vi "Scan Module.vi"(1 "Channel":u32(ring)=1 items=["A"=1, "B"=2, "A + B"=3, "C"=4, "A + C"=5, "A + B"=6, "D"=8, "A + D"=9, "B + D"=10, "C + D"=12, "A + B + C + D"=15], 9 "Init state":T1=enum."Init(GPU FFT)", 11 "Error In":errorcluster, 12 "Start Acquire?":bool) -> (4 "Finished?":bool, 15 "Error Out":errorcluster)   [LabVIEW 2018]
uses:
  Controls/Go Scan Actions.ctl
  Controls/FGV Actions.ctl
  Controls/Queue Manager Actions.ctl
  Controls/scan status.ctl
  Hardware Mfg/Thorlabs Translation Stages/Controls/Motion Translation Module Control.ctl
  Controls/Set Get Controls.ctl
  Tile naming actions.ctl
  Hardware Mfg/AlazarTech SDK/Controls/Alazar Engine Actions.ctl
  Controls/Save Bline to Mem Control.ctl
panel:
  out "Waveform Chart":dbl(graph)
  in  "No Slice?":bool
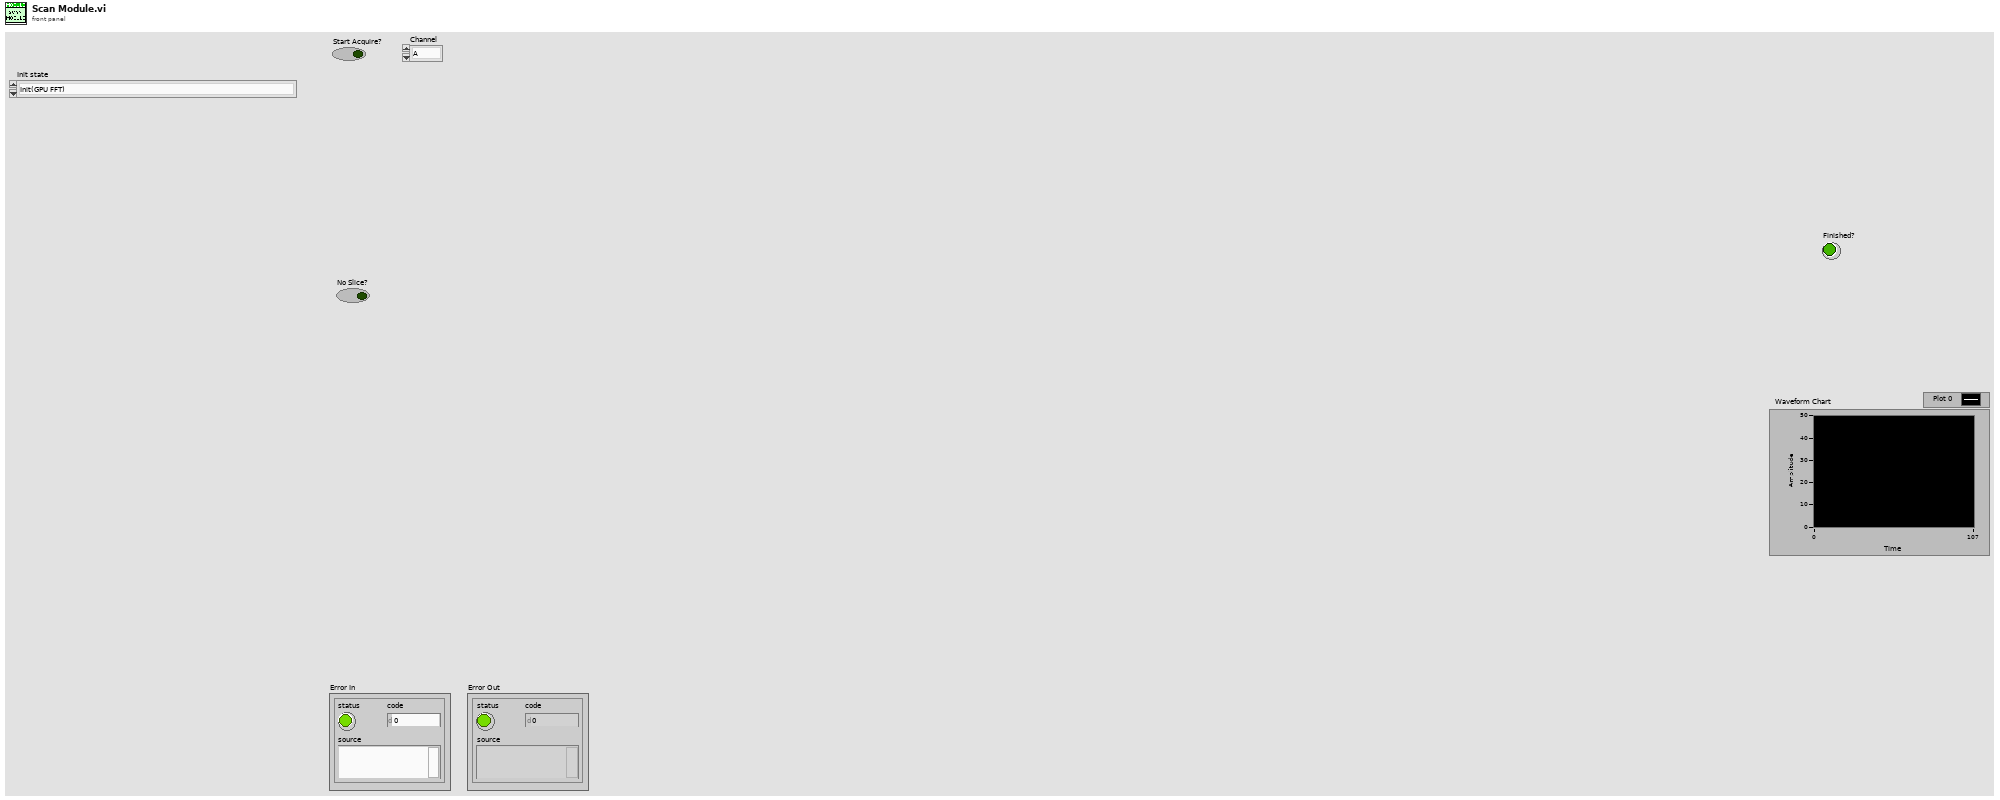
[diagram p1: front panel]
types:
  T1 = typedef "Go Scan Actions.ctl" = enum16{"Init(ThorOCT Spatial)", "Init(ThorOCT Spectral)", "Init(GPU FFT)", "Init(Alazar FFT)", "Init Scan Head(ThorOCT Spectral)", "Init Scan Head(ThorOCT Spatial)", "Init Scan Head", "Init Table Stage", "Init Vibratome", "Generate Mosaic", "Generate Z Position", "Go to Image Z", "Go Image Home", "Go Mosaic", "Acquire Image(ThorOCT Spatial)", "Acquire Image(ThorOCT Spectral)", "Acquire Image(GPU FFT)", "Acquire Image(Alazar FFT)", "Go Vibratome", "Slice", "Finished(ThorOCT)", "Finished", "Init(Alazar Spectral)"}
  T2 = typedef "FGV Actions.ctl" = enum16{"Init", "Set", "Get", "Clear"}
  T3 = typedef "System Parameters.ctl" = cluster{"Optical Parameters":T4, "Vibratome":T5, "Table Stages":T6, "Imaging Parameter":T9, "Galvo HW Parameters":cluster{"Analog Out Channel":tag, "Min Voltage":dbl, "Max Voltage":dbl, "Pixel Clock Source":tag, "Sample Rate":dbl, "Line Clock Out Ch":tag}, "Alazar parameters":T11, "Mosaic Paramter":cluster{"X Axis":cluster{"Start [mm]":dbl, "Steps [pts]":dbl, "End [mm]":dbl}, "Y Axis":cluster{"Start [mm]":dbl, "Steps [pts]":dbl, "End [mm]":dbl}, "Scan Pattern":enum16{"Uni-directional", "Bi-Directional", "Spiral Out", "Spiral In"}, "Overlap Options":cluster{"Overlap Type":enum16{"No Overlap", "X Only", "Y Only", "X and Y"}, "Percent Overlap":u8, "Justify":enum16{"Start", "Center", "End"}}}, "Manual Controls":T18, "Vibratome Axis":T21}
  T4 = typedef "Optical Parameters.ctl" = cluster{"Obj. Focal Length [mm]":dbl, "Scan Lens EFL[mm]":dbl, "Tube Lens EFL[mm]":dbl, "Galvo V Range (+/-)":dbl, "Galvo Max Half Angle [Deg]":dbl, "Max Galvo Range[%]":dbl}
  T5 = typedef "Vibratome Parameters.ctl" = cluster{"Z Bottom [mm]":dbl, "Pre Cut Dwell [s]":dbl, "Blade Frequency [RPM]":u16, "Slice Speed [mm/s]":dbl, "Post Cut Dwell [s]":dbl, "Ramp Time [s]":dbl, "Start X [mm]":dbl, "Start Y [mm]":dbl, "Slice Length [mm]":dbl, "Slice Axis":enum16{"X Axis", "Y Axis", "Z Axis"}, "Controller VISA Ref":refnum<visa-resource-name>}
  T6 = typedef "Translation Stage Parameters.ctl" = cluster{"X Stage":T7, "Y Stage":T7, "Z Stage":T7}
  T7 = typedef "Translation Stage Cluster.ctl" = cluster{"Position":dbl, "Is.Enabled?":bool, "Is.Connected?":bool, "Device SN":string, "AccelerationMaximum":dbl, "VelocityMaximum":dbl, "Acceleration":dbl, "Velocity":dbl, "waitTimeout (ms)":i32, "Model":T8, "Is.Homed?":bool}
  T8 = typedef "Translation Stage Types.ctl" = enum16{"None", "Thorlabs LTS", "Thorlabs MLJ"}
  T9 = typedef "Imaging Parameters.ctl" = cluster{"Raster Scan Direction":T10, "Pixel Dwell Time [Clock Cycles]":u16, "Flyback Time [Clock Cycles]":u16, "XY Center [um]":cluster{"X":dbl, "Y":dbl}, "Pixel Step Size [um] X":dbl, "XY Image Size":enum16{"32 x 32", "64 x 64", "128 x 128", "256 x 256", "512 x 512", "1024 x 1024", "2048 x 2048"}, "Custom":bool, "Custom Size":cluster{"X":u16, "Y":u16}, "Line Averages":u8, "Pixel Step Size [um] Y":dbl}
  T10 = typedef "Scan Direction.ctl" = enum16{"Uni Directional", "Bi Directional", "None"}
  T11 = typedef "Alazar parameters.ctl" = cluster{"Trigger Settings":cluster{"General Trigger Settings":T12, "Trigger Engine 1":T13, "Trigger Engine 2":T13}, "Device ID":T14, "Ch A Input Control":T15, "Ch B Input Control":T15, "Acq Settings":T16, "Capture Clock":T17}
  T12 = typedef "General Trigger Settings.ctl" = cluster{"Trigger Operation":u32, "Coupling ID":u32, "Range ID":u32, "Delay":u32, "Timeout Ticks":u32, "Mode":u32, "Parameter":u32}
  T13 = typedef "Trigger Engine Controls.ctl" = cluster{"Trigger Engine":u32, "Source":u32, "Slope":u32, "Level":u32}
  T14 = typedef "Alazar Device ID.ctl" = cluster{"System ID":u32, "Board ID":u32}
  T15 = typedef "Channel Input Controls.ctl" = cluster{"Channel":u8, "Coupling":u32, "Range":u32, "Impedance":u32}
  T16 = typedef "Alazar Acquisition Settings.ctl" = cluster{"Record Length":u32, "Offset":u32, "Records Per Buffer":u32, "Records Count (Records/Acq)":u32, "Window Type":u32, "Footer":u32, "Samples per record":u32, "Output Format":u32}
  T17 = typedef "Clock Controls.ctl" = cluster{"Sample Rate":u32, "Decimation":u32, "Source":u32, "Edge":u32}
  T18 = typedef "Manual Controls.ctl" = cluster{"Z0":dbl, "First image height":dbl, "Data Path":path, "Save parameters":T19, "Center Galvos":bool, "Acquisition mode":T20, "PSOCT Channel":u32, "Save":bool, "AIP rotation angle":dbl, "Scan Parameters":cluster{"# Scan":cluster{"#Ascan":i32, "#Bscan":i32}, "# Rpt":cluster{"#ARpt":i32, "#BRpt":i32}, "Aline Rate":u16, "# Extra":cluster{"# ARpt_extra":i32, "#Brtn_extra":i32}}, "ROI Parameters":cluster{"ROI (mm)":cluster{"X (mm)":dbl, "Y (mm)":dbl}, "Shift (mm)":cluster{"Xshift (mm)":sgl, "Yshift (mm)":sgl}}, "Objective":u16}
  T19 = typedef "FFT parameters.ctl" = cluster{"start pixel":i32, "#pixels to save":i32}
  T20 = typedef "FFT mode.ctl" = enum16{"ThorOCT B line", "ThorOCT Spectral", "ThorOCT FFT", "Alazar B line", "Alazar FFT", "GPU FFT", "Alazar Spectral"}
  T21 = typedef "Vibratome Param.ctl" = cluster{"Start [mm](first cut height)":dbl, "slice thickness[um]":dbl, "#slice":u16, "slice thick2[um]":dbl, "#thin slices":u16, "image thickness(um)":dbl, "#images":u16, "image depth2":dbl, "#image depth2":u16}
  T22 = typedef "Queue Manager Actions.ctl" = enum16{"Init", "Enqueue", "Enqueue All", "Preview Queue", "Dequeue", "Get Status", "Flush Queue", "Flush All Queues", "Release All Queues", "Release Queue", "Enqueue at Opposite End"}
  T23 = typedef "scan status.ctl" = enum16{"Complete Scan(ThorOCT)", "Complete Scan(PSOCT)", "Start(ThorOCT Spatial)", "Start(ThorOCT Spectral)", "Start(GPU FFT)", "Start(Alazar FFT)", "Scan(ThorOCT Spatial)", "Scan(ThorOCT Spectral)", "Scan(GPU FFT)", "Scan(Alazar FFT)", "Finish Scan(ThorOCT)", "Finish Scan(PSOCT)"}
  T24 = typedef "Set Get Controls.ctl" = enum16{"Set", "Get"}
  T25 = typedef "Motion Translation Module Control.ctl" = enum16{"Init", "Home", "Status", "Velocity/Accel", "Position", "Jog", "Stop", "Uninit", "Enable", "Disable"}
  T26 = typedef "Tile naming actions.ctl" = enum16{"Export", "Increment", "Total tile num", "Init"}
  T27 = typedef "Alazar Engine Actions.ctl" = enum16{"Init", "Config Clock", "Config Ch", "Config Trig", "Config Non-FFT Acq.", "Non-FFT Acquire", "start acquire", "Config Acq.", "Acquire", "UnInit"}
  T28 = enum16{"Configure channels", "Write Scan Pattern", "Start Galvo Task", "Is Task Done?", "Stop Galvo", "Uninit", "Init: Calc scan pattern"}
  T29 = enum16{"Init", "Configure", "Configure Data", "Generate Scan Pattern", "Start Acquire Raw", "Start Acquire Data", "Acquire RAW", "Acquire Data", "Stop Acquire", "Uninit"}
  T30 = typedef "Save Bline to Mem Control.ctl" = enum16{"Output data", "Save(ThorOCT)", "Save(PSOCT)", "FFT and Save", "Uninit", "PSOCT Spectral buffer Set", "PSOCT Spatial buffer Set", "PSOCT Spectral buffer Init", "PSOCT Spatial buffer Init", "ThorOCT Spectral buffer Init", "ThorOCT Spatial buffer Init", "ThorOCT Spectral buffer Set", "ThorOCT Spatial buffer Set", "ThorOCT Spectral Save", "Alazar Spectral Save"}
  T31 = typedef "ScanType.ctl" = enum16{"Single Frame", "Continuous Frame", "ROI Line", "Vibratome", "Mosaic", "Mosaic + Slice"}
  T32 = cluster{"X Axis":cluster{"Start [mm]":dbl, "Steps [pts]":dbl, "End [mm]":dbl}, "Y Axis":cluster{"Start [mm]":dbl, "Steps [pts]":dbl, "End [mm]":dbl}, "Scan Pattern":enum16{"Uni-directional", "Bi-Directional", "Spiral Out", "Spiral In"}, "Overlap Options":cluster{"Overlap Type":enum16{"No Overlap", "X Only", "Y Only", "X and Y"}, "Percent Overlap":u8, "Justify":enum16{"Start", "Center", "End"}}}
  T33 = cluster{"Start [mm]":dbl, "Steps [pts]":dbl, "End [mm]":dbl}
  T34 = cluster{"Overlap Type":enum16{"No Overlap", "X Only", "Y Only", "X and Y"}, "Percent Overlap":u8, "Justify":enum16{"Start", "Center", "End"}}
  T35 = enum16{"Uni-directional", "Bi-Directional", "Spiral Out", "Spiral In"}
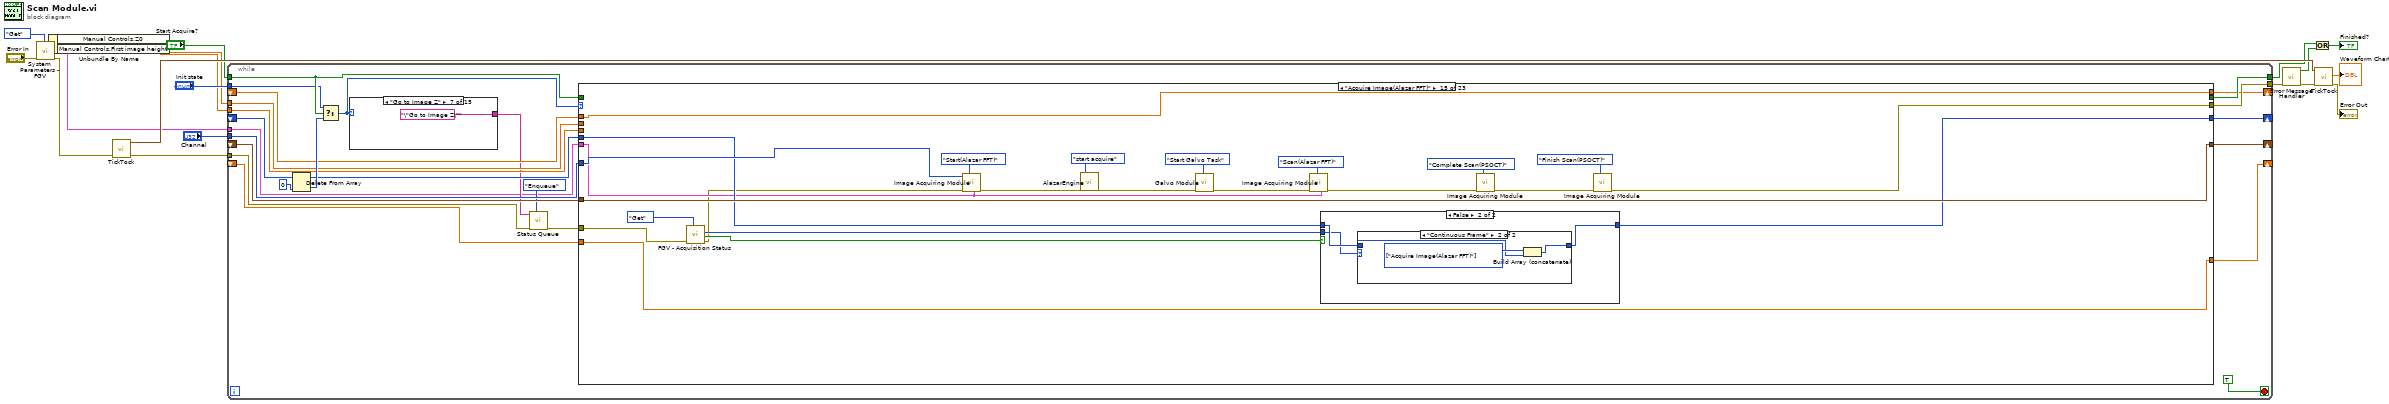
[diagram p0: block diagram]
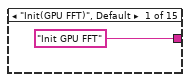
[diagram p2: hidden frame]
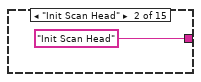
[diagram p3: hidden frame]
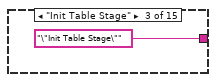
[diagram p4: hidden frame]
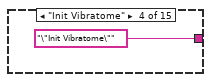
[diagram p5: hidden frame]
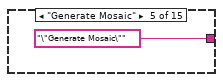
[diagram p6: hidden frame]
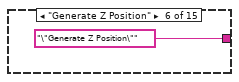
[diagram p7: hidden frame]
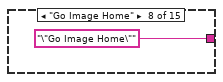
[diagram p8: hidden frame]
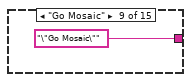
[diagram p9: hidden frame]
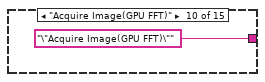
[diagram p10: hidden frame]
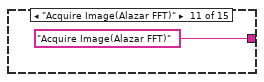
[diagram p11: hidden frame]
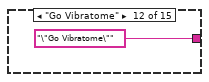
[diagram p12: hidden frame]
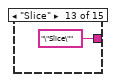
[diagram p13: hidden frame]
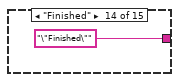
[diagram p14: hidden frame]
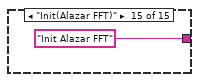
[diagram p15: hidden frame]
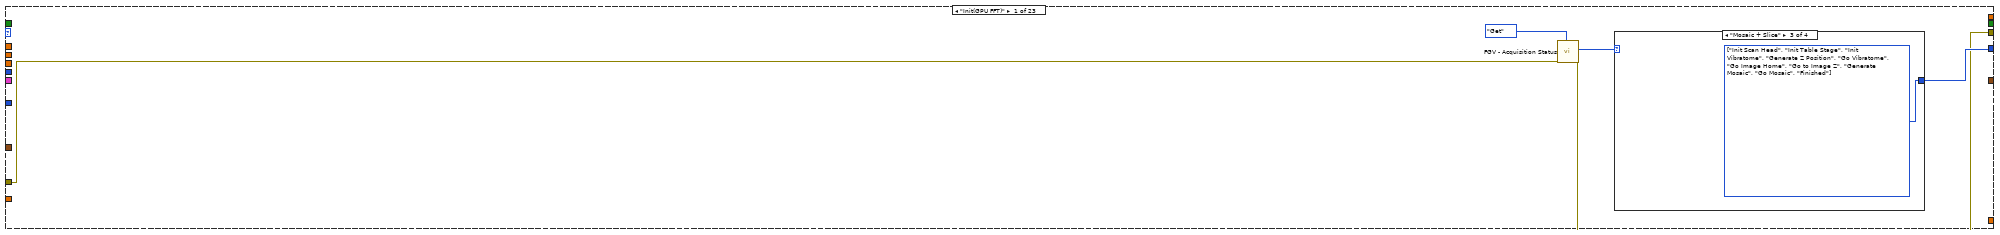
[diagram p16: hidden frame]
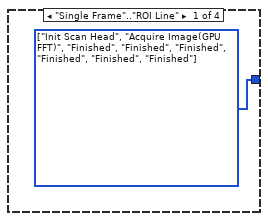
[diagram p17: hidden frame]
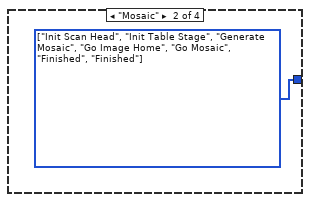
[diagram p18: hidden frame]
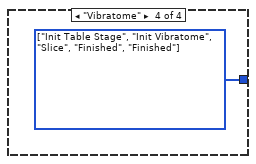
[diagram p19: hidden frame]
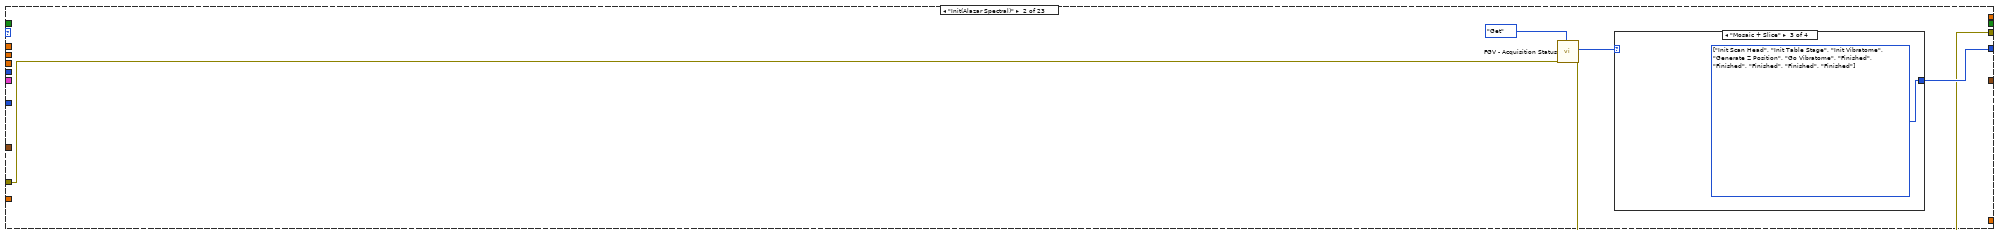
[diagram p20: hidden frame]
diagram:
  n1 = call "System Parameters - FGV.vi"("Actions"=FGV_Actions."Get", "Error In"="Error In") -> ("Error Out"=w4:errorcluster, "System Parameters [Out]"=w3:T3)  [unwired: 8 in]
  n2 = Unbundle By Name(w3) -> ("Manual Controls.Z0"=w2:dbl, "Manual Controls.First image height"=w1:dbl)
  n3 = call "TickTock.vi"("Error In"=w4) -> ("Error Out"=w16:errorcluster, "Current Time (Out)"=w14:timestamp)  [unwired: 8 in, 1 out]
  n4 = while {
    shift-right: [w37] -> _
    shift-left: _ -> [w42]
    tunnel: "Start Acquire?" -> [w38]
    shift-right: [w36] -> _
    shift-left: _ -> [w34]
    tunnel: w16 -> [w24]
    tunnel: [w35] -> w18
    tunnel: [w33] -> w10
    tunnel: w1 -> [w32]
    shift-right: [w30] -> _
    shift-left: _ -> [w28]
    shift-right: [w31] -> _
    shift-left: _ -> [w29]
    tunnel: "Init state" -> [w27]
    tunnel: w2 -> [w26]
    tunnel: "Channel" -> [w25]
    tunnel: w3 -> [w19]
    stop <- TRUE stop-if-true
    n5 = Delete From Array(array=w42, index=0) -> (deleted portion=w41:T1, array with subset deleted=w40:T1[])  [unwired: 1 in]
    n6 = Select(t=w27, s=w38, f=w41) -> (s? t:f=w22:T1)
    n7 = case shown="\"Go to Image Z\"" w22 {
      tunnel: ["Init GPU FFT" "Init Scan Head" "\"Init Table Stage\"" "\"Init Vibratome\"" "\"Generate Mosaic\"" "\"Generate Z Position\"" "\"Go to Image Z\"" "\"Go Image Home\"" "\"Go Mosaic\"" "\"Acquire Image(GPU FFT)\"" "Acquire Image(Alazar FFT)" "\"Go Vibratome\"" "\"Slice\"" "\"Finished\"" "Init Alazar FFT"] -> w21
      frame "Init(GPU FFT)", Default {
      }
      frame "Init Scan Head" {
      }
      frame "Init Table Stage" {
      }
      frame "Init Vibratome" {
      }
      frame "Generate Mosaic" {
      }
      frame "Generate Z Position" {
      }
      frame "Go to Image Z" {
      }
      frame "Go Image Home" {
      }
      frame "Go Mosaic" {
      }
      frame "Acquire Image(GPU FFT)" {
      }
      frame "Acquire Image(Alazar FFT)" {
      }
      frame "Go Vibratome" {
      }
      frame "Slice" {
      }
      frame "Finished" {
      }
      frame "Init(Alazar FFT)" {
      }
    }
    n8 = call "Status Queue.vi"("Action"=Queue_Manager_Actions."Enqueue", "Error In"=w24, "Status Message [In]"=w21) -> ("Error Out"=w23:errorcluster)  [unwired: 7 in, 1 out]
    n9 = case shown="\"Acquire Image(Alazar FFT)\"" w22 {
      selector: w22 -> [_ _ _ _ _ _ _ _ _ _ _ _ _ _ _ _ _ _ w397 _ _ _ _]
      tunnel: [w62 w71 w80 w89 w97 w118 w125 w133 w141 w172 w182 w198 w220 w232 w279 w311 w336 w364 w403 w465 w530 _ _] -> w37
      tunnel: w40 -> [_ _ _ _ _ w118 w125 w133 w141 w172 w182 w198 w220 w233 w282 w314 w339 w365 w405 w467 w532 _ _]
      tunnel: [_ _ _ _ _ w121 w126 w134 w142 w173 w183 w185 w231 w241 w295 w320 w345 w370 w406 w468 w533 _ _] -> w36
      tunnel: w34 -> [_ _ _ _ _ w121 w126 w134 w142 w173 w183 _ w231 w241 w295 w320 w345 w370 w402 w468 w533 _ _]
      tunnel: [w59 w68 w77 w86 w95 w119 w122 w129 w137 w171 w177 w186 w214 w240 w277 w305 w330 w358 w404 w466 w531 w550 w594] -> w35
      tunnel: w38 -> [_ _ _ _ _ _ _ _ _ _ _ _ _ _ _ _ _ _ _ _ _ _ _]
      tunnel: [_ _ _ _ _ _ _ _ _ _ _ _ _ _ _ _ _ _ _ _ w524 TRUE TRUE] -> w33
      tunnel: w32 -> [_ _ _ _ _ w111 _ _ _ _ _ _ _ _ _ _ _ _ _ _ _ _ _]
      tunnel: [_ _ _ _ _ w116 w123 w131 w139 w169 w181 w192 w216 w238 w286 w317 w342 w368 w395 w459 w523 _ _] -> w31
      tunnel: [_ _ _ _ _ w110 w124 w132 w140 w170 w180 w191 w215 w236 w285 w316 w341 w367 w393 w458 w527 _ _] -> w30
      tunnel: w29 -> [_ _ _ _ _ _ w123 w131 w139 w169 w181 w192 w216 w238 w286 w317 w342 w368 w395 w456 w523 _ _]
      tunnel: w28 -> [_ _ _ _ _ _ w124 w132 w140 w170 w180 w191 w215 w234 w285 w316 w341 w367 w393 w458 w527 _ _]
      tunnel: w23 -> [w60 w69 w78 w87 w96 w119 w122 w130 w138 w144 w178 w190 w200 w237 w275 w308 w333 w362 w394 w464 w529 w551 w595]
      tunnel: w26 -> [_ _ _ _ _ _ _ _ _ _ _ _ _ _ _ _ _ _ _ w463 w528 _ _]
      tunnel: w25 -> [_ _ _ _ _ _ _ _ _ _ _ _ _ _ w283 _ _ w366 _ _ _ _ _]
      tunnel: w19 -> [_ _ _ _ _ w120 _ w128 w136 w143 w176 w189 w199 w239 w273 w309 w334 w359 w396 w457 w526 w563 w607]
      frame "Init(GPU FFT)" {
        n10 = call "FGV - Acquisition Status.vi"("Actions"=FGV_Actions."Get", "Error In"=w60) -> ("Error Out"=w59:errorcluster, "Scan Type [Out]"=w61:T31)  [unwired: 5 in, 3 out]
        n11 = case shown="\"Mosaic + Slice\"" w61 {
          tunnel: [w64 w65 w66 w67] -> w62
          frame "Single Frame".."ROI Line" {
            w64 = T1[] [enum."Init Scan Head", enum."Acquire Image(GPU FFT)", enum."Finished", enum."Finished", enum."Finished", enum."Finished", enum."Finished", enum."Finished"] items=["Init(ThorOCT Spatial)", "Init(ThorOCT Spectral)", "Init(GPU FFT)", "Init(Alazar FFT)", "Init Scan Head(ThorOCT Spectral)", "Init Scan Head(ThorOCT Spatial)", "Init Scan Head", "Init Table Stage", "Init Vibratome", "Generate Mosaic", "Generate Z Position", "Go to Image Z", "Go Image Home", "Go Mosaic", "Acquire Image(ThorOCT Spatial)", "Acquire Image(ThorOCT Spectral)", "Acquire Image(GPU FFT)", "Acquire Image(Alazar FFT)", "Go Vibratome", "Slice", "Finished(ThorOCT)", "Finished", "Init(Alazar Spectral)"]
          }
          frame "Mosaic" {
            w65 = T1[] [enum."Init Scan Head", enum."Init Table Stage", enum."Generate Mosaic", enum."Go Image Home", enum."Go Mosaic", enum."Finished", enum."Finished"] items=["Init(ThorOCT Spatial)", "Init(ThorOCT Spectral)", "Init(GPU FFT)", "Init(Alazar FFT)", "Init Scan Head(ThorOCT Spectral)", "Init Scan Head(ThorOCT Spatial)", "Init Scan Head", "Init Table Stage", "Init Vibratome", "Generate Mosaic", "Generate Z Position", "Go to Image Z", "Go Image Home", "Go Mosaic", "Acquire Image(ThorOCT Spatial)", "Acquire Image(ThorOCT Spectral)", "Acquire Image(GPU FFT)", "Acquire Image(Alazar FFT)", "Go Vibratome", "Slice", "Finished(ThorOCT)", "Finished", "Init(Alazar Spectral)"]
          }
          frame "Mosaic + Slice" {
            w66 = T1[] [enum."Init Scan Head", enum."Init Table Stage", enum."Init Vibratome", enum."Generate Z Position", enum."Go Vibratome", enum."Go Image Home", enum."Go to Image Z", enum."Generate Mosaic", enum."Go Mosaic", enum."Finished"] items=["Init(ThorOCT Spatial)", "Init(ThorOCT Spectral)", "Init(GPU FFT)", "Init(Alazar FFT)", "Init Scan Head(ThorOCT Spectral)", "Init Scan Head(ThorOCT Spatial)", "Init Scan Head", "Init Table Stage", "Init Vibratome", "Generate Mosaic", "Generate Z Position", "Go to Image Z", "Go Image Home", "Go Mosaic", "Acquire Image(ThorOCT Spatial)", "Acquire Image(ThorOCT Spectral)", "Acquire Image(GPU FFT)", "Acquire Image(Alazar FFT)", "Go Vibratome", "Slice", "Finished(ThorOCT)", "Finished", "Init(Alazar Spectral)"]
          }
          frame "Vibratome" {
            w67 = T1[] [enum."Init Table Stage", enum."Init Vibratome", enum."Slice", enum."Finished", enum."Finished"] items=["Init(ThorOCT Spatial)", "Init(ThorOCT Spectral)", "Init(GPU FFT)", "Init(Alazar FFT)", "Init Scan Head(ThorOCT Spectral)", "Init Scan Head(ThorOCT Spatial)", "Init Scan Head", "Init Table Stage", "Init Vibratome", "Generate Mosaic", "Generate Z Position", "Go to Image Z", "Go Image Home", "Go Mosaic", "Acquire Image(ThorOCT Spatial)", "Acquire Image(ThorOCT Spectral)", "Acquire Image(GPU FFT)", "Acquire Image(Alazar FFT)", "Go Vibratome", "Slice", "Finished(ThorOCT)", "Finished", "Init(Alazar Spectral)"]
          }
        }
      }
      frame "Init(Alazar Spectral)" {
        n12 = call "FGV - Acquisition Status.vi"("Actions"=FGV_Actions."Get", "Error In"=w69) -> ("Error Out"=w68:errorcluster, "Scan Type [Out]"=w70:T31)  [unwired: 5 in, 3 out]
        n13 = case shown="\"Mosaic + Slice\"" w70 {
          tunnel: [w73 w74 w75 w76] -> w71
          frame "Single Frame".."ROI Line" {
            w73 = T1[] [enum."Init Scan Head", enum."Init Scan Head", enum."Acquire Image(GPU FFT)", enum."Finished", enum."Acquire Image(GPU FFT)", enum."Finished", enum."Acquire Image(GPU FFT)", enum."Finished"] items=["Init(ThorOCT Spatial)", "Init(ThorOCT Spectral)", "Init(GPU FFT)", "Init(Alazar FFT)", "Init Scan Head(ThorOCT Spectral)", "Init Scan Head(ThorOCT Spatial)", "Init Scan Head", "Init Table Stage", "Init Vibratome", "Generate Mosaic", "Generate Z Position", "Go to Image Z", "Go Image Home", "Go Mosaic", "Acquire Image(ThorOCT Spatial)", "Acquire Image(ThorOCT Spectral)", "Acquire Image(GPU FFT)", "Acquire Image(Alazar FFT)", "Go Vibratome", "Slice", "Finished(ThorOCT)", "Finished", "Init(Alazar Spectral)"]
          }
          frame "Mosaic" {
            w74 = T1[] [enum."Init Scan Head", enum."Init Table Stage", enum."Generate Mosaic", enum."Go Image Home", enum."Go Mosaic", enum."Finished", enum."Finished"] items=["Init(ThorOCT Spatial)", "Init(ThorOCT Spectral)", "Init(GPU FFT)", "Init(Alazar FFT)", "Init Scan Head(ThorOCT Spectral)", "Init Scan Head(ThorOCT Spatial)", "Init Scan Head", "Init Table Stage", "Init Vibratome", "Generate Mosaic", "Generate Z Position", "Go to Image Z", "Go Image Home", "Go Mosaic", "Acquire Image(ThorOCT Spatial)", "Acquire Image(ThorOCT Spectral)", "Acquire Image(GPU FFT)", "Acquire Image(Alazar FFT)", "Go Vibratome", "Slice", "Finished(ThorOCT)", "Finished", "Init(Alazar Spectral)"]
          }
          frame "Mosaic + Slice" {
            w75 = T1[] [enum."Init Scan Head", enum."Init Table Stage", enum."Init Vibratome", enum."Generate Z Position", enum."Go Vibratome", enum."Finished", enum."Finished", enum."Finished", enum."Finished", enum."Finished"] items=["Init(ThorOCT Spatial)", "Init(ThorOCT Spectral)", "Init(GPU FFT)", "Init(Alazar FFT)", "Init Scan Head(ThorOCT Spectral)", "Init Scan Head(ThorOCT Spatial)", "Init Scan Head", "Init Table Stage", "Init Vibratome", "Generate Mosaic", "Generate Z Position", "Go to Image Z", "Go Image Home", "Go Mosaic", "Acquire Image(ThorOCT Spatial)", "Acquire Image(ThorOCT Spectral)", "Acquire Image(GPU FFT)", "Acquire Image(Alazar FFT)", "Go Vibratome", "Slice", "Finished(ThorOCT)", "Finished", "Init(Alazar Spectral)"]
          }
          frame "Vibratome" {
            w76 = T1[] [enum."Init Table Stage", enum."Init Vibratome", enum."Slice", enum."Finished", enum."Finished"] items=["Init(ThorOCT Spatial)", "Init(ThorOCT Spectral)", "Init(GPU FFT)", "Init(Alazar FFT)", "Init Scan Head(ThorOCT Spectral)", "Init Scan Head(ThorOCT Spatial)", "Init Scan Head", "Init Table Stage", "Init Vibratome", "Generate Mosaic", "Generate Z Position", "Go to Image Z", "Go Image Home", "Go Mosaic", "Acquire Image(ThorOCT Spatial)", "Acquire Image(ThorOCT Spectral)", "Acquire Image(GPU FFT)", "Acquire Image(Alazar FFT)", "Go Vibratome", "Slice", "Finished(ThorOCT)", "Finished", "Init(Alazar Spectral)"]
          }
        }
      }
      frame "Init(ThorOCT Spatial)" {
        n14 = call "FGV - Acquisition Status.vi"("Actions"=FGV_Actions."Get", "Error In"=w78) -> ("Error Out"=w77:errorcluster, "Scan Type [Out]"=w79:T31)  [unwired: 5 in, 3 out]
        n15 = case shown="\"Single Frame\"..\"ROI Line\"" w79 {
          tunnel: [w82 w83 w84 w85] -> w80
          frame "Single Frame".."ROI Line" {
            w82 = T1[] [enum."Init Scan Head(ThorOCT Spatial)", enum."Acquire Image(ThorOCT Spatial)", enum."Finished(ThorOCT)", enum."Finished", enum."Acquire Image(GPU FFT)", enum."Finished", enum."Acquire Image(GPU FFT)", enum."Finished"] items=["Init(ThorOCT Spatial)", "Init(ThorOCT Spectral)", "Init(GPU FFT)", "Init(Alazar FFT)", "Init Scan Head(ThorOCT Spectral)", "Init Scan Head(ThorOCT Spatial)", "Init Scan Head", "Init Table Stage", "Init Vibratome", "Generate Mosaic", "Generate Z Position", "Go to Image Z", "Go Image Home", "Go Mosaic", "Acquire Image(ThorOCT Spatial)", "Acquire Image(ThorOCT Spectral)", "Acquire Image(GPU FFT)", "Acquire Image(Alazar FFT)", "Go Vibratome", "Slice", "Finished(ThorOCT)", "Finished", "Init(Alazar Spectral)"]
          }
          frame "Mosaic" {
            w83 = T1[] [enum."Init Scan Head(ThorOCT Spatial)", enum."Init Table Stage", enum."Generate Mosaic", enum."Go Image Home", enum."Go Mosaic", enum."Finished(ThorOCT)", enum."Finished"] items=["Init(ThorOCT Spatial)", "Init(ThorOCT Spectral)", "Init(GPU FFT)", "Init(Alazar FFT)", "Init Scan Head(ThorOCT Spectral)", "Init Scan Head(ThorOCT Spatial)", "Init Scan Head", "Init Table Stage", "Init Vibratome", "Generate Mosaic", "Generate Z Position", "Go to Image Z", "Go Image Home", "Go Mosaic", "Acquire Image(ThorOCT Spatial)", "Acquire Image(ThorOCT Spectral)", "Acquire Image(GPU FFT)", "Acquire Image(Alazar FFT)", "Go Vibratome", "Slice", "Finished(ThorOCT)", "Finished", "Init(Alazar Spectral)"]
          }
          frame "Mosaic + Slice" {
            w84 = T1[] [enum."Init Scan Head(ThorOCT Spatial)", enum."Init Table Stage", enum."Init Vibratome", enum."Generate Z Position", enum."Generate Mosaic", enum."Go Image Home", enum."Go Mosaic", enum."Go Vibratome", enum."Finished(ThorOCT)", enum."Finished"] items=["Init(ThorOCT Spatial)", "Init(ThorOCT Spectral)", "Init(GPU FFT)", "Init(Alazar FFT)", "Init Scan Head(ThorOCT Spectral)", "Init Scan Head(ThorOCT Spatial)", "Init Scan Head", "Init Table Stage", "Init Vibratome", "Generate Mosaic", "Generate Z Position", "Go to Image Z", "Go Image Home", "Go Mosaic", "Acquire Image(ThorOCT Spatial)", "Acquire Image(ThorOCT Spectral)", "Acquire Image(GPU FFT)", "Acquire Image(Alazar FFT)", "Go Vibratome", "Slice", "Finished(ThorOCT)", "Finished", "Init(Alazar Spectral)"]
          }
          frame "Vibratome" {
            w85 = T1[] [enum."Init Table Stage", enum."Init Vibratome", enum."Slice", enum."Finished(ThorOCT)", enum."Finished(ThorOCT)"] items=["Init(ThorOCT Spatial)", "Init(ThorOCT Spectral)", "Init(GPU FFT)", "Init(Alazar FFT)", "Init Scan Head(ThorOCT Spectral)", "Init Scan Head(ThorOCT Spatial)", "Init Scan Head", "Init Table Stage", "Init Vibratome", "Generate Mosaic", "Generate Z Position", "Go to Image Z", "Go Image Home", "Go Mosaic", "Acquire Image(ThorOCT Spatial)", "Acquire Image(ThorOCT Spectral)", "Acquire Image(GPU FFT)", "Acquire Image(Alazar FFT)", "Go Vibratome", "Slice", "Finished(ThorOCT)", "Finished", "Init(Alazar Spectral)"]
          }
        }
      }
      frame "Init(ThorOCT Spectral)" {
        n16 = call "FGV - Acquisition Status.vi"("Actions"=FGV_Actions."Get", "Error In"=w87) -> ("Error Out"=w86:errorcluster, "Scan Type [Out]"=w88:T31)  [unwired: 5 in, 3 out]
        n17 = case shown="\"Vibratome\"" w88 {
          tunnel: [w91 w92 w93 w94] -> w89
          frame "Single Frame".."ROI Line" {
            w91 = T1[] [enum."Init Scan Head(ThorOCT Spectral)", enum."Acquire Image(ThorOCT Spectral)", enum."Finished(ThorOCT)", enum."Finished", enum."Acquire Image(GPU FFT)", enum."Finished", enum."Acquire Image(GPU FFT)", enum."Finished"] items=["Init(ThorOCT Spatial)", "Init(ThorOCT Spectral)", "Init(GPU FFT)", "Init(Alazar FFT)", "Init Scan Head(ThorOCT Spectral)", "Init Scan Head(ThorOCT Spatial)", "Init Scan Head", "Init Table Stage", "Init Vibratome", "Generate Mosaic", "Generate Z Position", "Go to Image Z", "Go Image Home", "Go Mosaic", "Acquire Image(ThorOCT Spatial)", "Acquire Image(ThorOCT Spectral)", "Acquire Image(GPU FFT)", "Acquire Image(Alazar FFT)", "Go Vibratome", "Slice", "Finished(ThorOCT)", "Finished", "Init(Alazar Spectral)"]
          }
          frame "Mosaic" {
            w92 = T1[] [enum."Init Scan Head(ThorOCT Spectral)", enum."Init Table Stage", enum."Generate Mosaic", enum."Go Image Home", enum."Go Mosaic", enum."Finished(ThorOCT)", enum."Finished"] items=["Init(ThorOCT Spatial)", "Init(ThorOCT Spectral)", "Init(GPU FFT)", "Init(Alazar FFT)", "Init Scan Head(ThorOCT Spectral)", "Init Scan Head(ThorOCT Spatial)", "Init Scan Head", "Init Table Stage", "Init Vibratome", "Generate Mosaic", "Generate Z Position", "Go to Image Z", "Go Image Home", "Go Mosaic", "Acquire Image(ThorOCT Spatial)", "Acquire Image(ThorOCT Spectral)", "Acquire Image(GPU FFT)", "Acquire Image(Alazar FFT)", "Go Vibratome", "Slice", "Finished(ThorOCT)", "Finished", "Init(Alazar Spectral)"]
          }
          frame "Mosaic + Slice" {
            w93 = T1[] [enum."Init Scan Head(ThorOCT Spectral)", enum."Init Table Stage", enum."Init Vibratome", enum."Generate Z Position", enum."Generate Mosaic", enum."Go Image Home", enum."Go Mosaic", enum."Go Vibratome", enum."Finished(ThorOCT)", enum."Finished"] items=["Init(ThorOCT Spatial)", "Init(ThorOCT Spectral)", "Init(GPU FFT)", "Init(Alazar FFT)", "Init Scan Head(ThorOCT Spectral)", "Init Scan Head(ThorOCT Spatial)", "Init Scan Head", "Init Table Stage", "Init Vibratome", "Generate Mosaic", "Generate Z Position", "Go to Image Z", "Go Image Home", "Go Mosaic", "Acquire Image(ThorOCT Spatial)", "Acquire Image(ThorOCT Spectral)", "Acquire Image(GPU FFT)", "Acquire Image(Alazar FFT)", "Go Vibratome", "Slice", "Finished(ThorOCT)", "Finished", "Init(Alazar Spectral)"]
          }
          frame "Vibratome" {
            w94 = T1[] [enum."Init Table Stage", enum."Init Vibratome", enum."Slice", enum."Finished(ThorOCT)", enum."Finished(ThorOCT)"] items=["Init(ThorOCT Spatial)", "Init(ThorOCT Spectral)", "Init(GPU FFT)", "Init(Alazar FFT)", "Init Scan Head(ThorOCT Spectral)", "Init Scan Head(ThorOCT Spatial)", "Init Scan Head", "Init Table Stage", "Init Vibratome", "Generate Mosaic", "Generate Z Position", "Go to Image Z", "Go Image Home", "Go Mosaic", "Acquire Image(ThorOCT Spatial)", "Acquire Image(ThorOCT Spectral)", "Acquire Image(GPU FFT)", "Acquire Image(Alazar FFT)", "Go Vibratome", "Slice", "Finished(ThorOCT)", "Finished", "Init(Alazar Spectral)"]
          }
        }
      }
      frame "Init(Alazar FFT)" {
        n18 = call "FGV - Acquisition Status.vi"("Actions"=FGV_Actions."Get", "Error In"=w96) -> ("Error Out"=w95:errorcluster, "Scan Type [Out]"=w98:T31)  [unwired: 5 in, 3 out]
        n19 = case shown="\"Mosaic + Slice\"" w98 {
          tunnel: [w100 w101 w102 w103 w104] -> w97
          frame "Single Frame", Default {
            w100 = T1[] [enum."Init Scan Head", enum."Acquire Image(Alazar FFT)", enum."Finished", enum."Finished", enum."Acquire Image(Alazar FFT)", enum."Finished", enum."Acquire Image(Alazar FFT)", enum."Finished"] items=["Init(ThorOCT Spatial)", "Init(ThorOCT Spectral)", "Init(GPU FFT)", "Init(Alazar FFT)", "Init Scan Head(ThorOCT Spectral)", "Init Scan Head(ThorOCT Spatial)", "Init Scan Head", "Init Table Stage", "Init Vibratome", "Generate Mosaic", "Generate Z Position", "Go to Image Z", "Go Image Home", "Go Mosaic", "Acquire Image(ThorOCT Spatial)", "Acquire Image(ThorOCT Spectral)", "Acquire Image(GPU FFT)", "Acquire Image(Alazar FFT)", "Go Vibratome", "Slice", "Finished(ThorOCT)", "Finished", "Init(Alazar Spectral)"]
          }
          frame "Continuous Frame" {
            w101 = T1[] [enum."Init Scan Head", enum."Acquire Image(Alazar FFT)", enum."Finished", enum."Finished", enum."Acquire Image(Alazar FFT)", enum."Finished", enum."Acquire Image(Alazar FFT)", enum."Finished"] items=["Init(ThorOCT Spatial)", "Init(ThorOCT Spectral)", "Init(GPU FFT)", "Init(Alazar FFT)", "Init Scan Head(ThorOCT Spectral)", "Init Scan Head(ThorOCT Spatial)", "Init Scan Head", "Init Table Stage", "Init Vibratome", "Generate Mosaic", "Generate Z Position", "Go to Image Z", "Go Image Home", "Go Mosaic", "Acquire Image(ThorOCT Spatial)", "Acquire Image(ThorOCT Spectral)", "Acquire Image(GPU FFT)", "Acquire Image(Alazar FFT)", "Go Vibratome", "Slice", "Finished(ThorOCT)", "Finished", "Init(Alazar Spectral)"]
          }
          frame "Mosaic" {
            w102 = T1[] [enum."Init Scan Head", enum."Init Table Stage", enum."Generate Mosaic", enum."Go Image Home", enum."Go Mosaic", enum."Finished", enum."Finished"] items=["Init(ThorOCT Spatial)", "Init(ThorOCT Spectral)", "Init(GPU FFT)", "Init(Alazar FFT)", "Init Scan Head(ThorOCT Spectral)", "Init Scan Head(ThorOCT Spatial)", "Init Scan Head", "Init Table Stage", "Init Vibratome", "Generate Mosaic", "Generate Z Position", "Go to Image Z", "Go Image Home", "Go Mosaic", "Acquire Image(ThorOCT Spatial)", "Acquire Image(ThorOCT Spectral)", "Acquire Image(GPU FFT)", "Acquire Image(Alazar FFT)", "Go Vibratome", "Slice", "Finished(ThorOCT)", "Finished", "Init(Alazar Spectral)"]
          }
          frame "Mosaic + Slice" {
            w103 = T1[] [enum."Init Scan Head", enum."Init Table Stage", enum."Init Vibratome", enum."Generate Z Position", enum."Go Vibratome", enum."Finished"] items=["Init(ThorOCT Spatial)", "Init(ThorOCT Spectral)", "Init(GPU FFT)", "Init(Alazar FFT)", "Init Scan Head(ThorOCT Spectral)", "Init Scan Head(ThorOCT Spatial)", "Init Scan Head", "Init Table Stage", "Init Vibratome", "Generate Mosaic", "Generate Z Position", "Go to Image Z", "Go Image Home", "Go Mosaic", "Acquire Image(ThorOCT Spatial)", "Acquire Image(ThorOCT Spectral)", "Acquire Image(GPU FFT)", "Acquire Image(Alazar FFT)", "Go Vibratome", "Slice", "Finished(ThorOCT)", "Finished", "Init(Alazar Spectral)"]
          }
          frame "Vibratome" {
            w104 = T1[] [enum."Init Table Stage", enum."Init Vibratome", enum."Slice", enum."Finished", enum."Finished"] items=["Init(ThorOCT Spatial)", "Init(ThorOCT Spectral)", "Init(GPU FFT)", "Init(Alazar FFT)", "Init Scan Head(ThorOCT Spectral)", "Init Scan Head(ThorOCT Spatial)", "Init Scan Head", "Init Table Stage", "Init Vibratome", "Generate Mosaic", "Generate Z Position", "Go to Image Z", "Go Image Home", "Go Mosaic", "Acquire Image(ThorOCT Spatial)", "Acquire Image(ThorOCT Spectral)", "Acquire Image(GPU FFT)", "Acquire Image(Alazar FFT)", "Go Vibratome", "Slice", "Finished(ThorOCT)", "Finished", "Init(Alazar Spectral)"]
          }
        }
      }
      frame "Generate Z Position" {
        w109 = 0.0
        w113 = 0.0 ("y")
        n20 = Unbundle By Name(w120) -> ("Vibratome Axis"=w117:T21)
        n21 = Unbundle By Name(w117) -> ("image thickness(um)"=w107:dbl, "#images"=w105:u16)
        n22 = Unbundle By Name(w117) -> ("Start [mm](first cut height)"=w115:dbl, "slice thickness[um]"=w114:dbl, "#slice"=w112:u16)
        n23 = Multiply(x=w112, y=w105) -> (x*y=w106:u16)
        n24 = call "Generate Z stage Position Aarray.vi"("#rep1"=w106, "#rep2"=w113, "thickness2"=w113, "Start Z"=w115, "thickness1"=w114) -> ("Array"=w116:dbl[])  [unwired: 6 in]
        n25 = Decrement(x=w105) -> (x-1=w108:u16)
        n26 = call "Generate Z stage Position Aarray.vi"("#rep1"=w108, "#rep2"=w109, "thickness2"=w109, "Start Z"=w111, "thickness1"=w107) -> ("Array"=w110:dbl[])  [unwired: 6 in]
      }
      frame "Init Scan Head" {
      }
      frame "Init Scan Head(ThorOCT Spatial)" {
        n27 = call "Image Acquiring Module.vi"("System Parameters"=w128, "Scan Status in"=scan_status."Start(ThorOCT Spatial)" ("Scan Status in 2"), "Error in"=w130) -> ("Error Out"=w129:errorcluster)  [unwired: 8 in]
      }
      frame "Init Scan Head(ThorOCT Spectral)" {
        n28 = call "Image Acquiring Module.vi"("System Parameters"=w136, "Scan Status in"=scan_status."Start(ThorOCT Spectral)" ("Scan Status in 2"), "Error in"=w138) -> ("Error Out"=w137:errorcluster)  [unwired: 8 in]
      }
      frame "Init Table Stage" {
        n29 = Unbundle By Name(w143) -> ("Table Stages"=w145:T6)
        n30 = call "XYZ Table Stage Module.vi"("Set/Get"=Set_Get_Controls."Set", "Action"=Motion_Translation_Module_Control."Init", "Error In"=w144, "Axis"=enum16{"X Axis", "Y Axis", "Z Axis"}."X Axis", "Table Stages"=w145) -> ("Error Out"=w167:errorcluster)  [unwired: 5 in, 1 out]
        n31 = call "XYZ Table Stage Module.vi"("Set/Get"=Set_Get_Controls."Set", "Action"=Motion_Translation_Module_Control."Init", "Error In"=w167, "Axis"=enum16{"X Axis", "Y Axis", "Z Axis"}."Y Axis", "Table Stages"=w145) -> ("Error Out"=w160:errorcluster)  [unwired: 5 in, 1 out]
        n32 = call "XYZ Table Stage Module.vi"("Set/Get"=Set_Get_Controls."Set", "Action"=Motion_Translation_Module_Control."Init", "Error In"=w160, "Axis"=enum16{"X Axis", "Y Axis", "Z Axis"}."Z Axis", "Table Stages"=w145) -> ("Error Out"=w146:errorcluster)  [unwired: 5 in, 1 out]
        n33 = call "XYZ Table Stage Module.vi"("Set/Get"=Set_Get_Controls."Set", "Action"=Motion_Translation_Module_Control."Velocity/Accel", "Error In"=w146, "Axis"=enum16{"X Axis", "Y Axis", "Z Axis"}."X Axis", "Table Stages"=w145) -> ("Error Out"=w156:errorcluster)  [unwired: 5 in, 1 out]
        n34 = call "XYZ Table Stage Module.vi"("Set/Get"=Set_Get_Controls."Set", "Action"=Motion_Translation_Module_Control."Velocity/Accel", "Error In"=w156, "Axis"=enum16{"X Axis", "Y Axis", "Z Axis"}."Y Axis", "Table Stages"=w145) -> ("Error Out"=w149:errorcluster)  [unwired: 5 in, 1 out]
        n35 = call "XYZ Table Stage Module.vi"("Set/Get"=Set_Get_Controls."Set", "Action"=Motion_Translation_Module_Control."Velocity/Accel", "Error In"=w149, "Axis"=enum16{"X Axis", "Y Axis", "Z Axis"}."Z Axis", "Table Stages"=w145) -> ("Error Out"=w171:errorcluster)  [unwired: 5 in, 1 out]
      }
      frame "Init Vibratome" {
        n36 = Unbundle By Name(w176) -> ("Table Stages"=w175:T6, "Vibratome"=w174:T5)
        n37 = call "Slice Engine.vi"("Table Stages"=w175, "error in (no error)"=w178, "Vibratome"=w174, "Action"="Configure Vibratome HW") -> ("error out"=w177:errorcluster)  [unwired: 7 in]
      }
      frame "Generate Mosaic" {
        n38 = Unbundle By Name(w189) -> ("Mosaic Paramter"=w193:T32)
        n39 = Unbundle By Name(w193) -> ("X Axis"=w197:T33, "Y Axis"=w196:T33, "Overlap Options"=w195:T34, "Scan Pattern"=w194:T35)
        n40 = call "Calculate X Y Step Size.vi"("Overlap Options"=w195, "Scan Pattern"=w194, "Error In"=w190, "Y Axis"=w196, "X Axis"=w197) -> ("Error Out"=w187:errorcluster, "Array"=w185:cluster{"X":dbl, "Y":dbl}[])  [unwired: 3 in, 2 out]
        n41 = Array Size(array=w185) -> (size(s)=w184:i32)
        n42 = call "Tile naming.vi"(7:Tile_naming_actions."Total tile num", "Error In"=w187, "Tile Num"=w184) -> ("Error Out"=w186:errorcluster)  [unwired: 6 in, 2 out]
      }
      frame "Go Image Home" {
        n43 = Unbundle By Name(w199) -> ("Mosaic Paramter"=w230:T32)
        n44 = Unbundle By Name(w230) -> ("X Axis"=w229:T33, "Y Axis"=w228:T33)
        n45 = Unbundle By Name(w229) -> ("End [mm]"=w218:dbl)
        n46 = Unbundle By Name(w228) -> ("End [mm]"=w217:dbl)
        n47 = Unbundle By Name(w199) -> ("Table Stages"=w219:T6)
        n48 = Bundle By Name(cluster=w219, "X Stage.Position"=w218, "Y Stage.Position"=w217) -> (w201:T6)
        n49 = call "XYZ Table Stage Module.vi"("Set/Get"=Set_Get_Controls."Set", "Action"=Motion_Translation_Module_Control."Velocity/Accel", "Error In"=w200, "Axis"=enum16{"X Axis", "Y Axis", "Z Axis"}."X Axis", "Table Stages"=w201) -> ("Error Out"=w212:errorcluster)  [unwired: 5 in, 1 out]
        n50 = call "XYZ Table Stage Module.vi"("Set/Get"=Set_Get_Controls."Set", "Action"=Motion_Translation_Module_Control."Velocity/Accel", "Error In"=w212, "Axis"=enum16{"X Axis", "Y Axis", "Z Axis"}."Y Axis", "Table Stages"=w201) -> ("Error Out"=w205:errorcluster)  [unwired: 5 in, 1 out]
        n51 = call "XYZ Table Stage Module.vi"("Set/Get"=Set_Get_Controls."Set", "Action"=Motion_Translation_Module_Control."Velocity/Accel", "Error In"=w205, "Axis"=enum16{"X Axis", "Y Axis", "Z Axis"}."Z Axis", "Table Stages"=w201) -> ("Error Out"=w202:errorcluster)  [unwired: 5 in, 1 out]
        n52 = call "XYZ Table Stage Module.vi"("Set/Get"=Set_Get_Controls."Set", "Action"=Motion_Translation_Module_Control."Position", "Error In"=w202, "Axis"=enum16{"X Axis", "Y Axis", "Z Axis"}."X Axis", "Table Stages"=w201) -> ("Error Out"=w221:errorcluster)  [unwired: 5 in, 1 out]
        n53 = call "XYZ Table Stage Module.vi"("Set/Get"=Set_Get_Controls."Set", "Action"=Motion_Translation_Module_Control."Position", "Error In"=w221, "Axis"=enum16{"X Axis", "Y Axis", "Z Axis"}."Y Axis", "Table Stages"=w201) -> ("Error Out"=w214:errorcluster)  [unwired: 5 in, 1 out]
      }
      frame "Go to Image Z" {
        n54 = Empty Array?(array=w234) -> (empty?=w235:bool)
        n55 = case shown="True" w235 {
          tunnel: [w243 w258] -> w240
          tunnel: w239 -> [_ w255]
          tunnel: w237 -> [w243 w251]
          tunnel: w234 -> [w244 w249]
          tunnel: [w244 w248] -> w236
          tunnel: w233 -> [_ w246]
          tunnel: [w242 w246] -> w232
          frame True {
            w242 = T1[] [enum."Finished"] items=["Init(ThorOCT Spatial)", "Init(ThorOCT Spectral)", "Init(GPU FFT)", "Init(Alazar FFT)", "Init Scan Head(ThorOCT Spectral)", "Init Scan Head(ThorOCT Spatial)", "Init Scan Head", "Init Table Stage", "Init Vibratome", "Generate Mosaic", "Generate Z Position", "Go to Image Z", "Go Image Home", "Go Mosaic", "Acquire Image(ThorOCT Spatial)", "Acquire Image(ThorOCT Spectral)", "Acquire Image(GPU FFT)", "Acquire Image(Alazar FFT)", "Go Vibratome", "Slice", "Finished(ThorOCT)", "Finished", "Init(Alazar Spectral)"]
          }
          frame False {
            n56 = flat-sequence {
              tunnel: w251 -> [w269]
              tunnel: [w263] -> w250
              tunnel: w247 -> [w262]
              frame #0 {
                # "update image plane"
                n57 = call "Scan engine status.vi"("Actions"=FGV_Actions."Get", "Error In"=w269) -> ("slice plane out"=w268:dbl, "XY Graph out"=w267:cluster{"X":dbl, "Y":dbl}[], "Current Position out"=w266:cluster{"X":dbl, "Y":dbl}, "Current state out"=w265:T1, "Error Out"=w264:errorcluster)  [unwired: 8 in, 1 out]
                n58 = call "Scan engine status.vi"("XY Graph in"=w267, "Actions"=FGV_Actions."Set", "Current Position in"=w266, "Current state in"=w265, "Error In"=w264, "image plane"=w262, "slice plane"=w268) -> ("Error Out"=w263:errorcluster)  [unwired: 3 in, 5 out]
              }
            }
            n59 = Delete From Array(array=w249, length=1, index=0) -> (deleted portion=w245:dbl[], array with subset deleted=w248:dbl[])
            n60 = Index Array(array=w245, index=0) -> (element=w247:dbl)
            n61 = Unbundle By Name(w255) -> ("Table Stages"=w257:T6)
            n62 = Bundle By Name(cluster=w257, "Z Stage.Position"=w247) -> (w256:T6)
            n63 = call "XYZ Table Stage Module.vi"("Set/Get"=Set_Get_Controls."Set", "Action"=Motion_Translation_Module_Control."Position", "Error In"=w250, "Axis"=enum16{"X Axis", "Y Axis", "Z Axis"}."Z Axis", "Table Stages"=w256) -> ("Error Out"=w258:errorcluster)  [unwired: 5 in, 1 out]
          }
        }
      }
      frame "Acquire Image(Alazar FFT)" {
        n64 = call "FGV - Acquisition Status.vi"("Actions"=FGV_Actions."Get", "Error In"=w275) -> ("Error Out"=w272:errorcluster, "Quit status out"=w276:bool, "Scan Type [Out]"=w280:T31)  [unwired: 5 in, 2 out]
        n65 = call "Image Acquiring Module.vi"("System Parameters"=w273, "Scan Status in"=scan_status."Start(Alazar FFT)" ("Scan Status in 2"), "Error in"=w272, "Channel"=w283) -> ("Error Out"=w287:errorcluster)  [unwired: 7 in]
        n66 = call "AlazarEngine.vi"("error in (no error)"=w287, "Action"=Alazar_Engine_Actions."start acquire") -> ("error out"=w290:errorcluster)  [unwired: 15 in, 2 out]
        n67 = call "Galvo Module.vi"("Action"=T28."Start Galvo Task", "error in (no error)"=w290) -> ("error out"=w294:errorcluster)  [unwired: 8 in, 1 out]
        n68 = call "Image Acquiring Module.vi"("System Parameters"=w273, "Scan Status in"=scan_status."Scan(Alazar FFT)", "Error in"=w294) -> ("Error Out"=w284:errorcluster)  [unwired: 8 in]
        n69 = case shown="False" w276 {
          tunnel: w282 -> [w296 w299]
          tunnel: w280 -> [_ w298]
          tunnel: [w296 w297] -> w279
          frame True {
          }
          frame False {
            n70 = case shown="\"Continuous Frame\"" w298 {
              tunnel: w299 -> [w300 w301]
              tunnel: [w300 w303] -> w297
              frame "Single Frame", Default {
              }
              frame "Continuous Frame" {
                w302 = T1[] [enum."Acquire Image(Alazar FFT)"] items=["Init(ThorOCT Spatial)", "Init(ThorOCT Spectral)", "Init(GPU FFT)", "Init(Alazar FFT)", "Init Scan Head(ThorOCT Spectral)", "Init Scan Head(ThorOCT Spatial)", "Init Scan Head", "Init Table Stage", "Init Vibratome", "Generate Mosaic", "Generate Z Position", "Go to Image Z", "Go Image Home", "Go Mosaic", "Acquire Image(ThorOCT Spatial)", "Acquire Image(ThorOCT Spectral)", "Acquire Image(GPU FFT)", "Acquire Image(Alazar FFT)", "Go Vibratome", "Slice", "Finished(ThorOCT)", "Finished", "Init(Alazar Spectral)"]
                n71 = Build Array (concatenate)(w302, w301) -> (w303:T1[])
              }
            }
          }
        }
        n72 = call "Image Acquiring Module.vi"("Scan Status in"=scan_status."Complete Scan(PSOCT)" ("Scan Status in 2"), "Error in"=w284) -> ("Error Out"=w278:errorcluster)  [unwired: 9 in]
        n73 = call "Image Acquiring Module.vi"("Scan Status in"=scan_status."Finish Scan(PSOCT)", "Error in"=w278) -> ("Error Out"=w277:errorcluster)  [unwired: 9 in]
      }
      frame "Acquire Image(ThorOCT Spectral)" {
        n74 = call "FGV - Acquisition Status.vi"("Actions"=FGV_Actions."Get", "Error In"=w308) -> ("Error Out"=w304:errorcluster, "Quit status out"=w310:bool, "Scan Type [Out]"=w312:T31)  [unwired: 5 in, 2 out]
        n75 = case shown="False" w310 {
          tunnel: w314 -> [w321 w324]
          tunnel: w312 -> [_ w323]
          tunnel: [w321 w322] -> w311
          frame True {
          }
          frame False {
            n76 = case shown="\"Continuous Frame\"" w323 {
              tunnel: w324 -> [w325 w326]
              tunnel: [w325 w328] -> w322
              frame "Single Frame", Default {
              }
              frame "Continuous Frame" {
                w327 = T1[] [enum."Acquire Image(ThorOCT Spectral)"] items=["Init(ThorOCT Spatial)", "Init(ThorOCT Spectral)", "Init(GPU FFT)", "Init(Alazar FFT)", "Init Scan Head(ThorOCT Spectral)", "Init Scan Head(ThorOCT Spatial)", "Init Scan Head", "Init Table Stage", "Init Vibratome", "Generate Mosaic", "Generate Z Position", "Go to Image Z", "Go Image Home", "Go Mosaic", "Acquire Image(ThorOCT Spatial)", "Acquire Image(ThorOCT Spectral)", "Acquire Image(GPU FFT)", "Acquire Image(Alazar FFT)", "Go Vibratome", "Slice", "Finished(ThorOCT)", "Finished", "Init(Alazar Spectral)"]
                n77 = Build Array (concatenate)(w327, w326) -> (w328:T1[])
              }
            }
          }
        }
        n78 = call "Thorlabs Module.vi"("Actions"=T29."Start Acquire Raw", "error in"=w304) -> ("error out"=w307:errorcluster)  [unwired: 6 in, 3 out]
        n79 = call "Image Acquiring Module.vi"("System Parameters"=w309, "Scan Status in"=scan_status."Scan(ThorOCT Spectral)", "Error in"=w307) -> ("Error Out"=w315:errorcluster)  [unwired: 8 in]
        n80 = call "Image Acquiring Module.vi"("Scan Status in"=scan_status."Complete Scan(ThorOCT)" ("Scan Status in 2"), "Error in"=w315) -> ("Error Out"=w305:errorcluster)  [unwired: 9 in]
      }
      frame "Acquire Image(ThorOCT Spatial)" {
        n81 = call "FGV - Acquisition Status.vi"("Actions"=FGV_Actions."Get", "Error In"=w333) -> ("Error Out"=w329:errorcluster, "Quit status out"=w335:bool, "Scan Type [Out]"=w337:T31)  [unwired: 5 in, 2 out]
        n82 = case shown="False" w335 {
          tunnel: w339 -> [w346 w349]
          tunnel: w337 -> [_ w348]
          tunnel: [w346 w347] -> w336
          frame True {
          }
          frame False {
            n83 = case shown="\"Continuous Frame\"" w348 {
              tunnel: w349 -> [w350 w351]
              tunnel: [w350 w353] -> w347
              frame "Single Frame", Default {
              }
              frame "Continuous Frame" {
                w352 = T1[] [enum."Acquire Image(ThorOCT Spatial)"] items=["Init(ThorOCT Spatial)", "Init(ThorOCT Spectral)", "Init(GPU FFT)", "Init(Alazar FFT)", "Init Scan Head(ThorOCT Spectral)", "Init Scan Head(ThorOCT Spatial)", "Init Scan Head", "Init Table Stage", "Init Vibratome", "Generate Mosaic", "Generate Z Position", "Go to Image Z", "Go Image Home", "Go Mosaic", "Acquire Image(ThorOCT Spatial)", "Acquire Image(ThorOCT Spectral)", "Acquire Image(GPU FFT)", "Acquire Image(Alazar FFT)", "Go Vibratome", "Slice", "Finished(ThorOCT)", "Finished", "Init(Alazar Spectral)"]
                n84 = Build Array (concatenate)(w352, w351) -> (w353:T1[])
              }
            }
          }
        }
        n85 = call "Thorlabs Module.vi"("Actions"=T29."Start Acquire Data", "error in"=w329) -> ("error out"=w332:errorcluster)  [unwired: 6 in, 3 out]
        n86 = call "Image Acquiring Module.vi"("System Parameters"=w334, "Scan Status in"=scan_status."Scan(ThorOCT Spatial)", "Error in"=w332) -> ("Error Out"=w340:errorcluster)  [unwired: 8 in]
        n87 = call "Image Acquiring Module.vi"("Scan Status in"=scan_status."Complete Scan(ThorOCT)" ("Scan Status in 2"), "Error in"=w340) -> ("Error Out"=w330:errorcluster)  [unwired: 9 in]
      }
      frame "Acquire Image(GPU FFT)" {
        n88 = call "FGV - Acquisition Status.vi"("Actions"=FGV_Actions."Get", "Error In"=w362) -> ("Error Out"=w354:errorcluster, "Quit status out"=w360:bool, "Scan Type [Out]"=w361:T31)  [unwired: 5 in, 2 out]
        n89 = case shown="False" w360 {
          tunnel: w365 -> [w384 w387]
          tunnel: w361 -> [_ w386]
          tunnel: [w384 w385] -> w364
          frame True {
          }
          frame False {
            n90 = case shown="\"Continuous Frame\"" w386 {
              tunnel: w387 -> [w388 w390]
              tunnel: [w388 w392] -> w385
              frame "Single Frame", Default {
              }
              frame "Continuous Frame" {
                w391 = T1[] [enum."Acquire Image(GPU FFT)"] items=["Init(ThorOCT Spatial)", "Init(ThorOCT Spectral)", "Init(GPU FFT)", "Init(Alazar FFT)", "Init Scan Head(ThorOCT Spectral)", "Init Scan Head(ThorOCT Spatial)", "Init Scan Head", "Init Table Stage", "Init Vibratome", "Generate Mosaic", "Generate Z Position", "Go to Image Z", "Go Image Home", "Go Mosaic", "Acquire Image(ThorOCT Spatial)", "Acquire Image(ThorOCT Spectral)", "Acquire Image(GPU FFT)", "Acquire Image(Alazar FFT)", "Go Vibratome", "Slice", "Finished(ThorOCT)", "Finished", "Init(Alazar Spectral)"]
                n91 = Build Array (concatenate)(w391, w390) -> (w392:T1[])
                n92 = Wait (ms)(milliseconds to wait=u32 1100) -> ()  [unwired: 1 out]
              }
            }
          }
        }
        n93 = call "Image Acquiring Module.vi"("System Parameters"=w359, "Scan Status in"=scan_status."Start(GPU FFT)" ("Scan Status in 2"), "Error in"=w354, "Channel"=w366) -> ("Error Out"=w371:errorcluster)  [unwired: 7 in]
        n94 = call "AlazarEngine.vi"("error in (no error)"=w371, "Action"=Alazar_Engine_Actions."start acquire") -> ("error out"=w374:errorcluster)  [unwired: 15 in, 2 out]
        n95 = call "Galvo Module.vi"("Action"=T28."Start Galvo Task", "error in (no error)"=w374) -> ("error out"=w378:errorcluster)  [unwired: 8 in, 1 out]
        n96 = call "Image Acquiring Module.vi"("System Parameters"=w359, "Scan Status in"=scan_status."Scan(GPU FFT)", "Error in"=w378) -> ("Error Out"=w369:errorcluster)  [unwired: 8 in]
        n97 = call "Image Acquiring Module.vi"("Scan Status in"=scan_status."Complete Scan(PSOCT)" ("Scan Status in 2"), "Error in"=w369) -> ("Error Out"=w357:errorcluster)  [unwired: 9 in]
        n98 = call "Image Acquiring Module.vi"("Scan Status in"=scan_status."Finish Scan(PSOCT)" ("Scan Status in 2"), "Error in"=w357) -> ("Error Out"=w356:errorcluster)  [unwired: 9 in]
        n99 = disable-structure shown="Enabled" {
          disable-tunnel: [w382 w383] -> w358
          disable-tunnel: w356 -> [w379 w383]
          frame Disabled {
            n100 = call "Process status.vi"("Actions"=FGV_Actions."Set", "Error In"=w379, "Status In"=FALSE) -> ("Error Out"=w382:errorcluster)  [unwired: 7 in, 1 out]
          }
          frame Enabled {
          }
        }
      }
      frame "Go Mosaic" {
        n101 = Empty Array?(array=w402) -> (empty?=w401:bool)
        n102 = flat-sequence {
          tunnel: [w415] -> w400
          tunnel: w399 -> [w414]
          tunnel: w398 -> [w413]
          tunnel: w397 -> [w412]
          tunnel: w394 -> [w411]
          frame #0 {
            # "update XY stage position"
            n103 = call "Scan engine status.vi"("Actions"=FGV_Actions."Get", "Error In"=w411) -> ("slice plane out"=w407:dbl, "image plane out"=w408:dbl, "Error Out"=w410:errorcluster)  [unwired: 8 in, 3 out]
            n104 = call "Scan engine status.vi"("XY Graph in"=w413, "Actions"=FGV_Actions."Set", "Current Position in"=w414, "Current state in"=w412, "Error In"=w410, "image plane"=w408, "slice plane"=w407) -> ("Error Out"=w415:errorcluster)  [unwired: 3 in, 5 out]
          }
        }
        n105 = Delete From Array(array=w402) -> (deleted portion=w399:cluster{"X":dbl, "Y":dbl}, array with subset deleted=w398:cluster{"X":dbl, "Y":dbl}[])  [unwired: 2 in]
        n106 = case shown="True" w401 {
          tunnel: [w422 w455] -> w406
          tunnel: w398 -> [w422 w455]
          tunnel: w405 -> [w423 w453]
          tunnel: [w437 w451] -> w403
          tunnel: [w418 w454] -> w404
          tunnel: w399 -> [w421 _]
          tunnel: w400 -> [w417 w454]
          tunnel: w396 -> [w419 _]
          tunnel: w393 -> [_ _]
          frame False {
            n107 = Unbundle By Name(w419) -> ("Table Stages"=w429:T6, "Manual Controls.Acquisition mode"=w420:T20)
            n108 = Unbundle By Name(w421) -> ("X"=w428:dbl, "Y"=w427:dbl)
            n109 = Bundle By Name(cluster=w429, "X Stage.Position"=w428, "Y Stage.Position"=w427) -> (w426:T6)
            n110 = call "XYZ Table Stage Module.vi"("Set/Get"=Set_Get_Controls."Set", "Action"=Motion_Translation_Module_Control."Position", "Error In"=w417, "Axis"=enum16{"X Axis", "Y Axis", "Z Axis"}."X Axis", "Table Stages"=w426) -> ("Error Out"=w424:errorcluster)  [unwired: 5 in, 1 out]
            n111 = call "XYZ Table Stage Module.vi"("Set/Get"=Set_Get_Controls."Set", "Action"=Motion_Translation_Module_Control."Position", "Error In"=w417, "Axis"=enum16{"X Axis", "Y Axis", "Z Axis"}."Y Axis", "Table Stages"=w426) -> ("Error Out"=w425:errorcluster)  [unwired: 5 in, 1 out]
            n112 = Merge Errors(w424, w425) -> (w418:errorcluster)
            n113 = case shown="\"Alazar Spectral\"" w420 {
              tunnel: [w438 w439 w440 w441 w442 w443 w450] -> w436
              tunnel: w418 -> [_ _ _ _ _ w444 _]
              frame "Alazar FFT", Default {
                w438 = T1[] [enum."Acquire Image(Alazar FFT)", enum."Go Mosaic"] items=["Init(ThorOCT Spatial)", "Init(ThorOCT Spectral)", "Init(GPU FFT)", "Init(Alazar FFT)", "Init Scan Head(ThorOCT Spectral)", "Init Scan Head(ThorOCT Spatial)", "Init Scan Head", "Init Table Stage", "Init Vibratome", "Generate Mosaic", "Generate Z Position", "Go to Image Z", "Go Image Home", "Go Mosaic", "Acquire Image(ThorOCT Spatial)", "Acquire Image(ThorOCT Spectral)", "Acquire Image(GPU FFT)", "Acquire Image(Alazar FFT)", "Go Vibratome", "Slice", "Finished(ThorOCT)", "Finished", "Init(Alazar Spectral)"]
              }
              frame "Alazar B line" {
                w439 = T1[] [enum."Acquire Image(Alazar FFT)", enum."Go Mosaic"] items=["Init(ThorOCT Spatial)", "Init(ThorOCT Spectral)", "Init(GPU FFT)", "Init(Alazar FFT)", "Init Scan Head(ThorOCT Spectral)", "Init Scan Head(ThorOCT Spatial)", "Init Scan Head", "Init Table Stage", "Init Vibratome", "Generate Mosaic", "Generate Z Position", "Go to Image Z", "Go Image Home", "Go Mosaic", "Acquire Image(ThorOCT Spatial)", "Acquire Image(ThorOCT Spectral)", "Acquire Image(GPU FFT)", "Acquire Image(Alazar FFT)", "Go Vibratome", "Slice", "Finished(ThorOCT)", "Finished", "Init(Alazar Spectral)"]
              }
              frame "ThorOCT FFT" {
                w440 = T1[] [enum."Acquire Image(ThorOCT Spatial)", enum."Go Mosaic"] items=["Init(ThorOCT Spatial)", "Init(ThorOCT Spectral)", "Init(GPU FFT)", "Init(Alazar FFT)", "Init Scan Head(ThorOCT Spectral)", "Init Scan Head(ThorOCT Spatial)", "Init Scan Head", "Init Table Stage", "Init Vibratome", "Generate Mosaic", "Generate Z Position", "Go to Image Z", "Go Image Home", "Go Mosaic", "Acquire Image(ThorOCT Spatial)", "Acquire Image(ThorOCT Spectral)", "Acquire Image(GPU FFT)", "Acquire Image(Alazar FFT)", "Go Vibratome", "Slice", "Finished(ThorOCT)", "Finished", "Init(Alazar Spectral)"]
              }
              frame "ThorOCT Spectral" {
                w441 = T1[] [enum."Acquire Image(ThorOCT Spectral)", enum."Go Mosaic"] items=["Init(ThorOCT Spatial)", "Init(ThorOCT Spectral)", "Init(GPU FFT)", "Init(Alazar FFT)", "Init Scan Head(ThorOCT Spectral)", "Init Scan Head(ThorOCT Spatial)", "Init Scan Head", "Init Table Stage", "Init Vibratome", "Generate Mosaic", "Generate Z Position", "Go to Image Z", "Go Image Home", "Go Mosaic", "Acquire Image(ThorOCT Spatial)", "Acquire Image(ThorOCT Spectral)", "Acquire Image(GPU FFT)", "Acquire Image(Alazar FFT)", "Go Vibratome", "Slice", "Finished(ThorOCT)", "Finished", "Init(Alazar Spectral)"]
              }
              frame "ThorOCT B line" {
                w442 = T1[] [enum."Acquire Image(ThorOCT Spatial)", enum."Go Mosaic"] items=["Init(ThorOCT Spatial)", "Init(ThorOCT Spectral)", "Init(GPU FFT)", "Init(Alazar FFT)", "Init Scan Head(ThorOCT Spectral)", "Init Scan Head(ThorOCT Spatial)", "Init Scan Head", "Init Table Stage", "Init Vibratome", "Generate Mosaic", "Generate Z Position", "Go to Image Z", "Go Image Home", "Go Mosaic", "Acquire Image(ThorOCT Spatial)", "Acquire Image(ThorOCT Spectral)", "Acquire Image(GPU FFT)", "Acquire Image(Alazar FFT)", "Go Vibratome", "Slice", "Finished(ThorOCT)", "Finished", "Init(Alazar Spectral)"]
              }
              frame "Alazar Spectral" {
                w443 = T1[] [enum."Acquire Image(GPU FFT)", enum."Go Mosaic"] items=["Init(ThorOCT Spatial)", "Init(ThorOCT Spectral)", "Init(GPU FFT)", "Init(Alazar FFT)", "Init Scan Head(ThorOCT Spectral)", "Init Scan Head(ThorOCT Spatial)", "Init Scan Head", "Init Table Stage", "Init Vibratome", "Generate Mosaic", "Generate Z Position", "Go to Image Z", "Go Image Home", "Go Mosaic", "Acquire Image(ThorOCT Spatial)", "Acquire Image(ThorOCT Spectral)", "Acquire Image(GPU FFT)", "Acquire Image(Alazar FFT)", "Go Vibratome", "Slice", "Finished(ThorOCT)", "Finished", "Init(Alazar Spectral)"]
                n114 = disable-structure shown="Disabled" {
                  disable-tunnel: w444 -> [w445 _]
                  frame Disabled {
                    n115 = while {
                      tunnel: w445 -> [w446]
                      stop <- w448 stop-if-true
                      n116 = call "Process status.vi"("Actions"=FGV_Actions."Get", "Error In"=w446) -> ("Status Out"=w448:bool)  [unwired: 8 in, 1 out]
                      n117 = Wait (ms)(milliseconds to wait=u32 500) -> ()  [unwired: 1 out]
                    }
                  }
                  frame Enabled {
                  }
                }
              }
              frame "GPU FFT" {
                w450 = T1[] [enum."Acquire Image(GPU FFT)", enum."Go Mosaic"] items=["Init(ThorOCT Spatial)", "Init(ThorOCT Spectral)", "Init(GPU FFT)", "Init(Alazar FFT)", "Init Scan Head(ThorOCT Spectral)", "Init Scan Head(ThorOCT Spatial)", "Init Scan Head", "Init Table Stage", "Init Vibratome", "Generate Mosaic", "Generate Z Position", "Go to Image Z", "Go Image Home", "Go Mosaic", "Acquire Image(ThorOCT Spatial)", "Acquire Image(ThorOCT Spectral)", "Acquire Image(GPU FFT)", "Acquire Image(Alazar FFT)", "Go Vibratome", "Slice", "Finished(ThorOCT)", "Finished", "Init(Alazar Spectral)"]
              }
            }
            n118 = Build Array (concatenate)(w436, w423) -> (w437:T1[])
          }
          frame True {
            w452 = T1[] [enum."Go Vibratome", enum."Go Vibratome", enum."Go Vibratome", enum."Go Vibratome", enum."Go Vibratome", enum."Go Image Home", enum."Go to Image Z", enum."Generate Mosaic", enum."Go Mosaic"] items=["Init(ThorOCT Spatial)", "Init(ThorOCT Spectral)", "Init(GPU FFT)", "Init(Alazar FFT)", "Init Scan Head(ThorOCT Spectral)", "Init Scan Head(ThorOCT Spatial)", "Init Scan Head", "Init Table Stage", "Init Vibratome", "Generate Mosaic", "Generate Z Position", "Go to Image Z", "Go Image Home", "Go Mosaic", "Acquire Image(ThorOCT Spatial)", "Acquire Image(ThorOCT Spectral)", "Acquire Image(GPU FFT)", "Acquire Image(Alazar FFT)", "Go Vibratome", "Slice", "Finished(ThorOCT)", "Finished", "Init(Alazar Spectral)"]
            n119 = Build Array (concatenate)(w452, w453) -> (w451:T1[])
          }
        }
      }
      frame "Go Vibratome" {
        n120 = Empty Array?(array=w456) -> (empty?=w462:bool)
        n121 = Or(x="No Slice?", y=w462) -> (x .or. y?=w461:bool)
        n122 = case shown="False" w461 {
          tunnel: w467 -> [w469 w522]
          tunnel: [w469 w522] -> w465
          tunnel: [w474 w521] -> w466
          tunnel: w464 -> [w477 w521]
          tunnel: w463 -> [w480 _]
          tunnel: [w485 _] -> w459
          tunnel: w457 -> [w470 _]
          tunnel: w456 -> [w476 _]
          frame False {
            n123 = flat-sequence {
              tunnel: [w502] -> w485
              tunnel: w476 -> [w501]
              tunnel: [w493] -> w475
              frame #0 {
                n124 = Delete From Array(array=w501, length=1, index=0) -> (deleted portion=w498:dbl[], array with subset deleted=w502:dbl[])
                n125 = Index Array(array=w498, index=0) -> (element=w493:dbl)
                n126 = call "Scan engine status.vi"("Actions"=FGV_Actions."Get") -> ("image plane out"=w492:dbl, "XY Graph out"=w491:cluster{"X":dbl, "Y":dbl}[], "Current Position out"=w490:cluster{"X":dbl, "Y":dbl}, "Current state out"=w489:T1, "Error Out"=w494:errorcluster)  [unwired: 9 in, 1 out]
                n127 = call "Scan engine status.vi"("XY Graph in"=w491, "Actions"=FGV_Actions."Set", "Current Position in"=w490, "Current state in"=w489, "Error In"=w494, "image plane"=w492, "slice plane"=w493) -> ()  [unwired: 3 in, 6 out]
              }
            }
            n128 = Unbundle By Name(w470) -> ("Table Stages"=w472:T6, "Vibratome"=w473:T5)
            n129 = Bundle By Name(cluster=w472, "Z Stage.Position"=w480) -> (w471:T6)
            n130 = flat-sequence {
              tunnel: [w517] -> w488
              tunnel: w477 -> [w516]
              tunnel: w471 -> [w515]
              frame #0 {
                # "Go to Z0"
                n131 = call "XYZ Table Stage Module.vi"("Set/Get"=Set_Get_Controls."Set", "Action"=Motion_Translation_Module_Control."Position", "Error In"=w516, "Axis"=enum16{"X Axis", "Y Axis", "Z Axis"}."Z Axis", "Table Stages"=w515) -> ("Error Out"=w517:errorcluster)  [unwired: 5 in, 1 out]
              }
            }
            n132 = call "Slice Engine.vi"("Table Stages"=w472, "error in (no error)"=w488, "Vibratome"=w473, "Action"="Move Stage (XY)") -> ("error out"=w486:errorcluster)  [unwired: 7 in]
            n133 = flat-sequence {
              tunnel: w486 -> [w505]
              tunnel: [w504] -> w483
              tunnel: w478 -> [w503]
              frame #0 {
                # "Go to next cut height"
                n134 = call "XYZ Table Stage Module.vi"("Set/Get"=Set_Get_Controls."Set", "Action"=Motion_Translation_Module_Control."Position", "Error In"=w505, "Axis"=enum16{"X Axis", "Y Axis", "Z Axis"}."Z Axis", "Table Stages"=w503) -> ("Error Out"=w504:errorcluster)  [unwired: 5 in, 1 out]
              }
            }
            n135 = Bundle By Name(cluster=w472, "Z Stage.Position"=w475) -> (w478:T6)
            n136 = call "Slice Engine.vi"("Table Stages"=w472, "error in (no error)"=w483, "Vibratome"=w473, "Action"="Set Slice Speed") -> ("error out"=w481:errorcluster)  [unwired: 7 in]
            n137 = call "Slice Engine.vi"("Table Stages"=w472, "error in (no error)"=w481, "Vibratome"=w473, "Action"="Slice") -> ("error out"=w479:errorcluster)  [unwired: 7 in]
            n138 = flat-sequence {
              tunnel: w479 -> [w511]
              tunnel: [w510] -> w474
              tunnel: w471 -> [w509]
              frame #0 {
                (unwired) "GO to Z0"
                # "Go to Z0"
                n139 = call "XYZ Table Stage Module.vi"("Set/Get"=Set_Get_Controls."Set", "Action"=Motion_Translation_Module_Control."Position", "Error In"=w511, "Axis"=enum16{"X Axis", "Y Axis", "Z Axis"}."Z Axis", "Table Stages"=w509) -> ("Error Out"=w510:errorcluster)  [unwired: 5 in, 1 out]
              }
            }
          }
          frame True {
          }
        }
      }
      frame "Slice" {
        n140 = Empty Array?(array=w523) -> (empty?=w524:bool)
        n141 = case shown="False" FALSE {
          tunnel: w532 -> [w534 w546]
          tunnel: [w534 w546] -> w530
          tunnel: [w535 w545] -> w531
          tunnel: w529 -> [w537 w545]
          tunnel: w528 -> [_ _]
          tunnel: w526 -> [w538 _]
          frame False {
            n142 = Unbundle By Name(w538) -> ("Table Stages"=w540:T6, "Vibratome"=w539:T5)
            n143 = call "Slice Engine.vi"("Table Stages"=w540, "error in (no error)"=w537, "Vibratome"=w539, "Action"="Move Stage (XY)") -> ("error out"=w536:errorcluster)  [unwired: 7 in]
            n144 = call "Slice Engine.vi"("Table Stages"=w540, "error in (no error)"=w536, "Vibratome"=w539, "Action"="Set Slice Speed") -> ("error out"=w541:errorcluster)  [unwired: 7 in]
            n145 = call "Slice Engine.vi"("Table Stages"=w540, "error in (no error)"=w541, "Vibratome"=w539, "Action"="Slice") -> ("error out"=w535:errorcluster)  [unwired: 7 in]
          }
          frame True {
          }
        }
      }
      frame "Finished", Default {
        n146 = call "Slice Engine.vi"("error in (no error)"=w551, "Action"="Uninit") -> ("error out"=w553:errorcluster)  [unwired: 9 in]
        n147 = call "Image Acquiring Module.vi"("Scan Status in"=scan_status."Finish Scan(PSOCT)", "Error in"=w553) -> ("Error Out"=w561:errorcluster)  [unwired: 9 in]
        n148 = call "FGV - Acquisition Status.vi"("Actions"=FGV_Actions."Get", "Error In"=w561) -> ("Error Out"=w562:errorcluster, "Quit status out"=w556:bool, "Scan Type [Out]"=w558:T31, "mem loc out"=w555:i32)  [unwired: 5 in, 1 out]
        n149 = call "FGV - Acquisition Status.vi"("mem loc"=w555, "Actions"=FGV_Actions."Set", "Error In"=w562, "Quit status"=w556, "Scan Type [In]"=w558, "Level Status In"=FALSE ("Status In")) -> ("Error Out"=w548:errorcluster)  [unwired: 1 in, 4 out]
        n150 = disable-structure shown="Enabled" {
          disable-tunnel: w548 -> [w578 w581]
          disable-tunnel: [w577 w581] -> w547
          frame Enabled {
            n151 = flat-sequence {
              tunnel: w578 -> [w580]
              tunnel: [w580] -> w577
              frame #0 {
                n152 = Wait (ms)(milliseconds to wait=u32 3000) -> ()  [unwired: 1 out]
              }
            }
          }
          frame Disabled {
          }
        }
        n153 = disable-structure shown="Enabled" {
          disable-tunnel: [w585 w587] -> w549
          disable-tunnel: w547 -> [w582 w587]
          frame Enabled {
            n154 = call "Save bline to memory1.vi"("action"=Save_Bline_to_Mem_Control."Uninit", "error in"=w582) -> ("error out"=w586:errorcluster)  [unwired: 13 in]
            n155 = call "Save bline to memory2.vi"("action"=Save_Bline_to_Mem_Control."Uninit", "error in"=w586) -> ("error out"=w585:errorcluster)  [unwired: 13 in]
          }
          frame Disabled {
          }
        }
        n156 = Unbundle By Name(w563) -> ("Table Stages"=w564:T6)
        n157 = call "XYZ Table Stage Module.vi"("Set/Get"=Set_Get_Controls."Set", "Action"=Motion_Translation_Module_Control."Uninit", "Error In"=w549, "Axis"=enum16{"X Axis", "Y Axis", "Z Axis"}."X Axis", "Table Stages"=w564) -> ("Error Out"=w574:errorcluster)  [unwired: 5 in, 1 out]
        n158 = call "XYZ Table Stage Module.vi"("Set/Get"=Set_Get_Controls."Set", "Action"=Motion_Translation_Module_Control."Uninit", "Error In"=w574, "Axis"=enum16{"X Axis", "Y Axis", "Z Axis"}."Y Axis", "Table Stages"=w564) -> ("Error Out"=w567:errorcluster)  [unwired: 5 in, 1 out]
        n159 = call "XYZ Table Stage Module.vi"("Set/Get"=Set_Get_Controls."Set", "Action"=Motion_Translation_Module_Control."Uninit", "Error In"=w567, "Axis"=enum16{"X Axis", "Y Axis", "Z Axis"}."Z Axis", "Table Stages"=w564) -> ("Error Out"=w550:errorcluster)  [unwired: 5 in, 1 out]
      }
      frame "Finished(ThorOCT)" {
        n160 = call "Slice Engine.vi"("error in (no error)"=w595, "Action"="Uninit") -> ("error out"=w596:errorcluster)  [unwired: 9 in]
        n161 = call "Image Acquiring Module.vi"("Scan Status in"=scan_status."Finish Scan(ThorOCT)", "Error in"=w596) -> ("Error Out"=w605:errorcluster)  [unwired: 9 in]
        n162 = call "FGV - Acquisition Status.vi"("Actions"=FGV_Actions."Get", "Error In"=w605) -> ("Error Out"=w606:errorcluster, "Quit status out"=w600:bool, "Scan Type [Out]"=w602:T31, "mem loc out"=w599:i32)  [unwired: 5 in, 1 out]
        n163 = call "FGV - Acquisition Status.vi"("mem loc"=w599, "Actions"=FGV_Actions."Set", "Error In"=w606, "Quit status"=w600, "Scan Type [In]"=w602, "Level Status In"=FALSE ("Status In")) -> ("Error Out"=w589:errorcluster)  [unwired: 1 in, 4 out]
        n164 = flat-sequence {
          tunnel: w589 -> [w622]
          tunnel: [w622] -> w588
          frame #0 {
            n165 = Wait (ms)(milliseconds to wait=u32 2000) -> ()  [unwired: 1 out]
          }
        }
        n166 = call "Save bline to memory1.vi"("action"=Save_Bline_to_Mem_Control."Uninit", "error in"=w588) -> ("error out"=w593:errorcluster)  [unwired: 13 in]
        n167 = Unbundle By Name(w607) -> ("Table Stages"=w608:T6)
        n168 = call "Save bline to memory2.vi"("action"=Save_Bline_to_Mem_Control."Uninit", "error in"=w593) -> ("error out"=w590:errorcluster)  [unwired: 13 in]
        n169 = call "XYZ Table Stage Module.vi"("Set/Get"=Set_Get_Controls."Set", "Action"=Motion_Translation_Module_Control."Uninit", "Error In"=w590, "Axis"=enum16{"X Axis", "Y Axis", "Z Axis"}."X Axis", "Table Stages"=w608) -> ("Error Out"=w618:errorcluster)  [unwired: 5 in, 1 out]
        n170 = call "XYZ Table Stage Module.vi"("Set/Get"=Set_Get_Controls."Set", "Action"=Motion_Translation_Module_Control."Uninit", "Error In"=w618, "Axis"=enum16{"X Axis", "Y Axis", "Z Axis"}."Y Axis", "Table Stages"=w608) -> ("Error Out"=w611:errorcluster)  [unwired: 5 in, 1 out]
        n171 = call "XYZ Table Stage Module.vi"("Set/Get"=Set_Get_Controls."Set", "Action"=Motion_Translation_Module_Control."Uninit", "Error In"=w611, "Axis"=enum16{"X Axis", "Y Axis", "Z Axis"}."Z Axis", "Table Stages"=w608) -> ("Error Out"=w594:errorcluster)  [unwired: 5 in, 1 out]
      }
    }
  }
  n172 = call "Error Message Handler.vi"("Error In"=w18) -> ("Error Out"=w17:errorcluster, "T button?"=w11:bool)  [unwired: 9 in]
  n173 = Or(x=w10, y=w11) -> (x .or. y?=→"Finished?":bool)
  n174 = call "TickTock.vi"("Error In"=w17, "Current Time (In)"=w14) -> ("Error Out"=→"Error Out":errorcluster, "dt"=→"Waveform Chart":dbl)  [unwired: 7 in, 1 out]
